vi "Image Status.vi"() -> ()   [LabVIEW 2017]
panel:
  in  "State":enum16{"Idle", "Motion", "Image"}(ring)
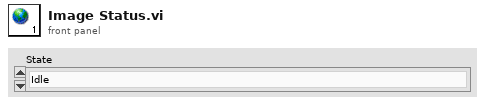
[diagram p1: front panel]
diagram:
